vi "RT Main.vi"() -> ()   [LabVIEW 2019]
doc: "The myRIO Project template acquires acceleration data from the onboard accelerometer and displays the changes of acceleration values in a waveform chart."
uses:
  <vilib>/Platform/TimedLoop/XDataNode/timing_clust.ctl
  <vilib>/Platform/TimedLoop/XDataNode/nitl_modes.ctl
  <vilib>/Platform/TimedLoop/XDataNode/wakeup.ctl
  <vilib>/myRIO/Instrument Drivers/Onboard IO/AI/typedefs/AI Reference.ctl
  <vilib>/myRIO/Common/Instrument Driver Framework/Utilities/typedefs/myRIO Generic Hardware Reference.ctl
  <vilib>/myRIO/Common/Instrument Driver Framework/Utilities/typedefs/Hardware Version Enum.ctl
  <vilib>/myRIO/Common/Instrument Driver Framework/Utilities/typedefs/myRIO v1.0 Reference.ctl
  <vilib>/myRIO/Common/Instrument Driver Framework/Utilities/typedefs/Generic FPGA Reference.ctl
  <vilib>/myRIO/Common/Instrument Driver Framework/myRIO v1.0/AI/typedefs/AI Channels List.ctl
  <vilib>/myRIO/Common/Instrument Driver Framework/myRIO v1.0/AI/typedefs/AI Channels Enum.ctl
  <vilib>/myRIO/Common/Instrument Driver Framework/Utilities/typedefs/Analog Scaling Constants List.ctl
  <vilib>/myRIO/Common/Instrument Driver Framework/Utilities/typedefs/Analog Scaling Constants.ctl
  <vilib>/userDefined/High Color/nirio_resource_hc.ctl
  <vilib>/Simulation/Shared/_Datatypes/SIM SISO Transfer Function.ctl
  <vilib>/Analysis/Matrix/Datatypes/RealMatrix.ctl
  <vilib>/myRIO/Instrument Drivers/Onboard IO/AO/typedefs/AO Reference.ctl
  <vilib>/myRIO/Common/Instrument Driver Framework/myRIO v1.0/AO/typedefs/AO Channels List.ctl
  <vilib>/myRIO/Common/Instrument Driver Framework/myRIO v1.0/AO/typedefs/AO Channels Enum.ctl
  <vilib>/myRIO/Common/Instrument Driver Framework/Utilities/vis/Is FPGA Ref Available.vi
  <vilib>/myRIO/Common/Instrument Driver Framework/myRIO v1.0/AI/vis/myRIO v1.1 Open AI.vi
  <vilib>/myRIO/Instrument Drivers/Onboard IO/AI/vis/Read.vi
  <vilib>/Simulation/DiscreteLinear/Implementation/NILVSim Discrete Transfer Function Direct.llb/SIM Discrete Transfer Function Diagram (SISO).vi
  <vilib>/Analysis/7linalg.llb/Real Transpose Matrix.vi
  <vilib>/Analysis/baseanly.llb/Real A x B.vi
  <vilib>/myRIO/Common/Instrument Driver Framework/myRIO v1.0/AO/vis/myRIO v1.1 Open AO.vi
  <vilib>/myRIO/Instrument Drivers/Onboard IO/AO/vis/Write.vi
  <vilib>/myRIO/Common/Instrument Driver Framework/Utilities/vis/Validate Channels.vi
  <vilib>/myRIO/Common/Instrument Driver Framework/myRIO v1.0/AI/vis/myRIO v1.0 Reserve AI.vi
  <vilib>/Simulation/ContinuousLinear/Implementation/Shared/SIM Transfer Function Support.llb/SIM TransferFunction Normalize to Buffer.vi
  <vilib>/Simulation/DiscreteLinear/Implementation/Shared/SIM Init Discrete States.vi
  <vilib>/Simulation/DiscreteLinear/Implementation/NILVSim Discrete Transfer Function Direct.llb/SIM Transfer Function Direct core (SISO).vi
  <vilib>/myRIO/Common/Instrument Driver Framework/myRIO v1.0/AO/vis/myRIO v1.0 Reserve AO.vi
  <vilib>/myRIO/Common/Instrument Driver Framework/myRIO v1.0/AI/vis/myRIO v1.0 Build MUX Configuration AI.vi
  <vilib>/myRIO/Common/Instrument Driver Framework/myRIO v1.0/Resource Manager/vis/myRIO v1.0 Reserve Channel List.vi
  <vilib>/Simulation/ContinuousLinear/Implementation/Shared/SIM Transfer Function Support.llb/SIM TransferFunction Normalize.vi
  <vilib>/myRIO/Common/Instrument Driver Framework/myRIO v1.0/AO/vis/myRIO v1.0 Build MUX Configuration AO.vi
  <vilib>/myRIO/Common/Instrument Driver Framework/myRIO v1.0/Resource Manager/vis/myRIO v1.0 Reserve Channel.vi
  <vilib>/myRIO/Common/Instrument Driver Framework/myRIO v1.0/Resource Manager/vis/myRIO v1.0 Unreserve Channel.vi
  <vilib>/Simulation/Implementation/Shared/SIM Polynomials.llb/SIM Remove Zero Coefficients (DBL).vi
  <vilib>/myRIO/Common/Instrument Driver Framework/myRIO v1.0/Resource Manager/vis/myRIO v1.0 Build Mutex Name.vi
  <vilib>/Utility/VariantDataType/GetNumericInfo.vi
  <vilib>/Utility/error.llb/Error Cluster From Error Code.vi
  <vilib>/myRIO/Common/Instrument Driver Framework/myRIO v1.0/myRIO v1.1 Open.vi
  <vilib>/myRIO/Common/Instrument Driver Framework/myRIO v1.0/AI/vis/myRIO v1.0 Get Scaling Constants AI.vi
  <vilib>/myRIO/Common/Instrument Driver Framework/Utilities/vis/IO Manager.vi
  <vilib>/myRIO/Common/Instrument Driver Framework/Utilities/vis/Configuration Manager.vi
  <vilib>/myRIO/Common/Instrument Driver Framework/myRIO v1.0/myRIO v1.0 Close.vi
  <vilib>/myRIO/Common/Instrument Driver Framework/myRIO v1.0/AI/vis/myRIO v1.0 Read AI.vi
  <vilib>/Simulation/Implementation/Shared/SIM Polynomials.llb/SIM Divide Polynomials (DBL).vi
  <vilib>/Simulation/Implementation/Shared/SIM BuildSimErr.vi
  <vilib>/Analysis/Matrix/Numeric/Multiply/Multiply - R,RM.vi
  <vilib>/Analysis/Matrix/Numeric/Conversions/Array To Matrix - RA.vi
  <vilib>/myRIO/Common/Instrument Driver Framework/myRIO v1.0/AO/vis/myRIO v1.0 Get Scaling Constants AO.vi
  <vilib>/myRIO/Common/Instrument Driver Framework/myRIO v1.0/AO/vis/myRIO v1.0 Write AO.vi
  <vilib>/platform/TimedLoop/XDataNode/XDataNode.xnode
  <vilib>/myRIO/Express VI/Onboard IO/AI/AI Express VI.xnode
  <vilib>/myRIO/Instrument Drivers/Onboard IO/AI/vis/myRIO AI Open.xnode
  <vilib>/Simulation/Implementation/XNodeFramework/SimXNode/SimX.xnode
  <vilib>/myRIO/Express VI/Onboard IO/AO/AO Express VI.xnode
  <vilib>/myRIO/Instrument Drivers/Onboard IO/AO/vis/myRIO AO Open.xnode
  <vilib>/myRIO/Instrument Drivers/Onboard IO/AO/AO.lvlib
  <vilib>/Analysis/Matrix/NI_Matrix.lvlib
  <vilib>/myRIO/Instrument Drivers/Onboard IO/AI/AI.lvlib
  <vilib>/gmath/NI_Gmath.lvlib
  <vilib>/Analysis/NI_AALPro.lvlib
  <vilib>/Analysis/NI_AALBase.lvlib
  <vilib>/Platform/TimedLoop/XDataNode/XDNodeRunTimeDep.lvlib
  <vilib>/ptbypt/NI_PtbyPt.lvlib
panel:
  out "j data":dbl[](array[numeric])
  out "u data":dbl[](array[numeric])
  out "dx data":dbl[](array[numeric])
  out "x data":dbl[](array[numeric])
  out "sucess":bool
  in  "amplitude":dbl=0.0003
  out "imp":dbl
  out "Exitation":dbl(graph)
  out "dt":dbl=0.0005
  out "PD":bool
  out "J":dbl
  out "run time[s]":dbl
  out "t":dbl
  in  "max J":dbl=10.0
  out "control_law":string
  out "iterations":i32
  out "Last Cost (J)":dbl
  out "iteration duration":i64(graph)
  out "u[A]":dbl(graph)
  out "x[um]":dbl(graph)
  in  "Stop EM":bool=TRUE
  in  "Stop Button":bool
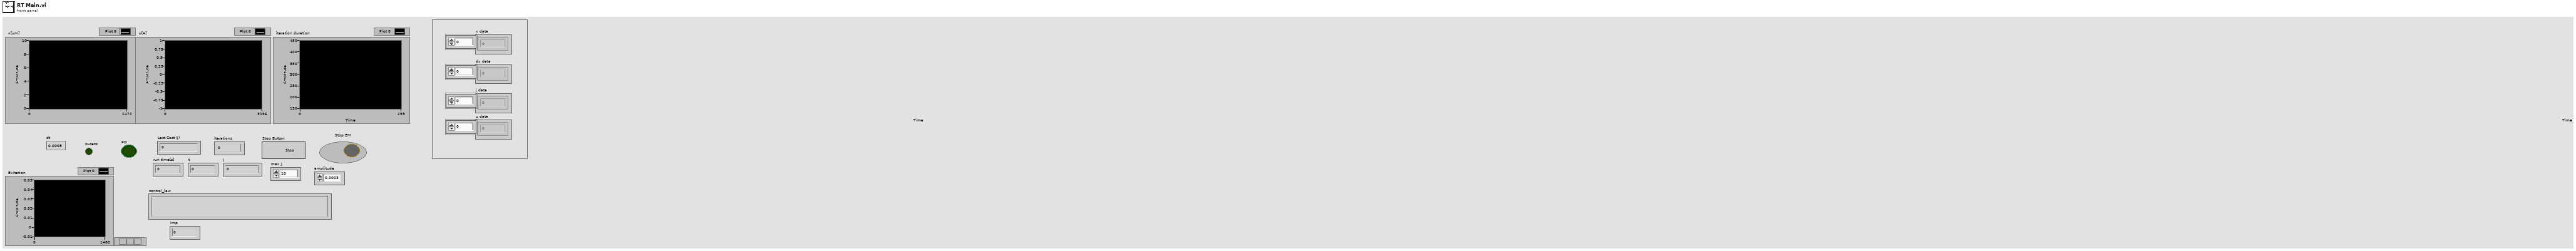
[diagram p1: front panel]
types:
  T1 = typedef "NI_Matrix.lvlib/RealMatrix.ctl" = dbl[][]
  T2 = typedef "SIM SISO Transfer Function.ctl" = cluster{"Numerator":dbl[], "Denominator":dbl[]}
  T3 = typedef "AO.lvlib/AO Reference.ctl" = cluster{"myRIO Reference":T4, "AO Channel List":T8, "AO Scaling Constant List":T10}
  T4 = typedef "myRIO Generic Hardware Reference.ctl" = cluster{"myRIO Model":T5, "myRIO Hardware Reference":T6}
  T5 = typedef "Hardware Version Enum.ctl" = enum16{"Unknown", "myRIO-1900", "myRIO-1950", "roboRIO", "NI ELVIS RIO CM", "ELVIS III"}
  T6 = typedef "myRIO v1.0 Reference.ctl" = cluster{"Generic FPGA Reference":T7, "Allow multiple opens":bool}
  T7 = typedef "Generic FPGA Reference.ctl" = refnum<k20>
  T8 = typedef "AO Channels List.ctl" = T9[]
  T9 = typedef "AO Channels Enum.ctl" = enum16{"Not Connected", "AudioOut/Left", "AudioOut/Right", "C/AO0", "C/AO1", "A/AO0", "A/AO1", "B/AO0", "B/AO1"}
  T10 = typedef "Analog Scaling Constants List.ctl" = T11[]
  T11 = typedef "Analog Scaling Constants.ctl" = cluster{"LSB Weight (Volts)":dbl, "Offset (Volts)":dbl, "Signed?":bool}
  T12 = typedef "nirio_resource_hc.ctl" = tag
  T13 = typedef "AI.lvlib/AI Reference.ctl" = cluster{"myRIO Reference":T4, "AI Channels List":T14, "AI Scaling Constants List":T10}
  T14 = typedef "AI Channels List.ctl" = T15[]
  T15 = typedef "AI Channels Enum.ctl" = enum16{"Not Connected", "AudioIn/Left", "AudioIn/Right", "C/AI0", "C/AI1", "A/AI0", "A/AI1", "A/AI2", "A/AI3", "A/AI4", "A/AI5", "A/AI6", "A/AI7", "B/AI0", "B/AI1", "B/AI2", "B/AI3", "B/AI4", "B/AI5", "B/AI6", "B/AI7", "AI/AI0", "AI/AI1", "AI/AI2", "AI/AI3", "A/AI0 (DIFF)", "A/AI1 (DIFF)", "A/AI2 (DIFF)", "A/AI3 (DIFF)", "B/AI0 (DIFF)", "B/AI1 (DIFF)", "B/AI2 (DIFF)", "B/AI3 (DIFF)"}
  T16 = typedef "XDNodeRunTimeDep.lvlib/timing_clust.ctl" = cluster{"Expected End [f-1]":u64, "Actual End [f-1]":u64, "Finished Late? [f-1]":bool, "Expected End [i-1]":u64, "Actual End [i-1]":u64, "Finished Late? [i-1]":bool, "Expected Start [i]":u64, "Actual Start [i]":u64, "Expected Start [f]":u64, "Actual Start [f]":u64, "Source Name":string, "Structure Name":string, "Period":i64, "Deadline":i64, "Offset":i64, "Start":i64, "Priority":i32, "Timeout":i32, "Mode":T17, "Wakeup Reason":T18, "Error":errorcluster, "Source Type":string, "Secondary Source Type":string, "Global End Time":u64, "Global Start Time":u64, "Frame Duration":u64, "Iteration Duration":u64, "Assigned CPU":i32, "I/O Scan Engine Mode":u32}
  T17 = typedef "XDNodeRunTimeDep.lvlib/nitl_modes.ctl" = enum32{"No Change", "Process missed periods, maintain original phase", "Discard missed periods, maintain original phase", "Process missed periods, ignore original phase", "Discard missed periods, ignore original phase"}
  T18 = typedef "XDNodeRunTimeDep.lvlib/wakeup.ctl" = enum32{"Normal", "Aborted", "Asynchronous wakeup", "Timing source error", "Timed loop error", "Timeout"}
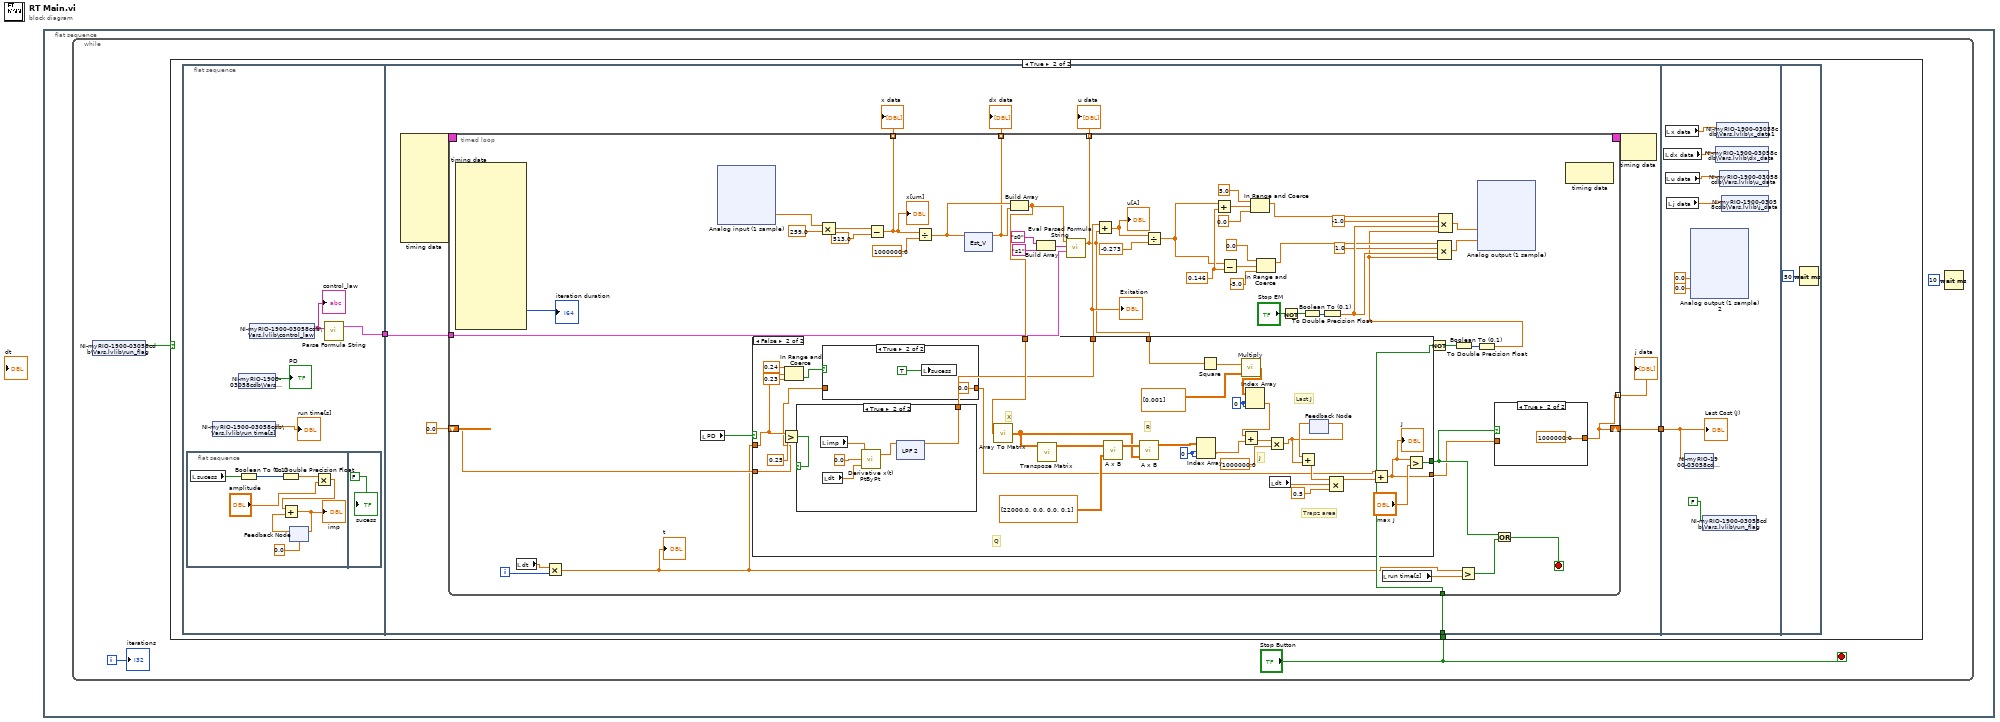
[diagram p0: block diagram]
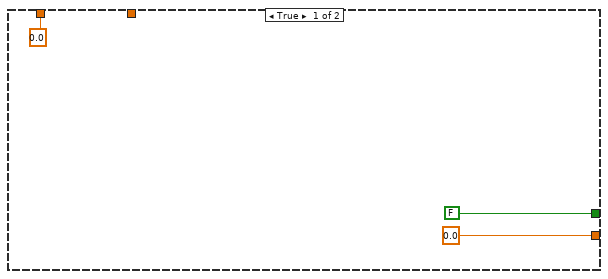
[diagram p4: hidden frame]
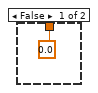
[diagram p6: hidden frame]
diagram:
  n1 = flat-sequence {
    frame #0 {
      n2 = while {
        i -> [w4]
        stop <- "Stop Button" stop-if-true
        n3 = shared-variable "NI-myRIO-1900-03058cdb\\Vars.lvlib\\run_flag"() -> (w2:bool)  [unwired: 1 in, 1 out]
        n4 = case shown="True" w2 {
          tunnel: "Stop Button" -> [_ w5]
          frame False {
          }
          frame True {
            n5 = flat-sequence {
              tunnel: [w10] -> w7
              tunnel: w7 -> [w28]
              tunnel: [w26] -> w6
              tunnel: w5 -> [w25]
              tunnel: w6 -> [w226]
              frame #0 {
                n6 = flat-sequence {
                  frame #0 {
                    n7 = local read "sucess"() -> (w17:bool)
                    n8 = Boolean To (0,1)(Boolean=w17) -> (0, 1=w18:i16)
                    n9 = To Double Precision Float(number=w18) -> (double precision float=w16:dbl)
                    n10 = feedback #1(0.0) -> (w19:dbl)
                    n11 = Multiply(x=w16, y="amplitude") -> (x*y=w12:dbl)
                    n12 = Add(x=w12, y=w19) -> (x+y=w13:dbl)
                    "imp" <- w13
                    n13 = feedback-in #1(w13) -> ()
                  }
                  frame #1 {
                    "sucess" <- FALSE ("sucess")
                  }
                }
                n14 = shared-variable "NI-myRIO-1900-03058cdb\\Vars.lvlib\\run time[s]"() -> (→"run time[s]":dbl)  [unwired: 1 in, 1 out]
                n15 = shared-variable "NI-myRIO-1900-03058cdb\\Vars.lvlib\\PD"() -> (→"PD":bool)  [unwired: 1 in, 1 out]
                n16 = shared-variable "NI-myRIO-1900-03058cdb\\Vars.lvlib\\control_law"() -> (w11:string)  [unwired: 1 in, 1 out]
                "control_law" <- w11
                n17 = call <vilib>:"Parse Formula String.vi"("formula"=w11) -> ("Parsed Formula"=w10:cluster{"Table":i32[][], "Y Values":dbl[]})  [unwired: 1 in, 1 out]
              }
              frame #1 {
                n18 = node-c288() -> (w30:T16)  [unwired: 10 in]
                n19 = timed-loop {
                  timing: w30 -> [_]
                  timing-out: [_] -> w29
                  shift-right: [w32] -> w26
                  shift-left: 0.0 -> [w59]
                  tunnel: w28 -> [w58]
                  tunnel: w25 -> [w41]
                  tunnel: [w35] -> w24 mode=indexing
                  tunnel: [w34] -> w23 mode=indexing
                  tunnel: [w33] -> w22 mode=indexing
                  tunnel: [w32] -> w21 mode=indexing
                  i -> [w47]
                  stop <- w44 stop-if-true
                  w75 = 0.146 ("y")
                  n20 = node-c288() -> (→"iteration duration":i64)  [unwired: 1 in, 16 out]
                  n21 = local read "dt"() -> (w31:dbl)
                  n22 = Multiply(x=w31, y=w47) -> (x*y=w37:dbl)
                  "t" <- w37
                  n23 = local read "PD"() -> (w43:bool)
                  n24 = xnode "Analog input (1 sample)"() -> ("C/AI1 (AI1)"=w64:dbl)  [unwired: 1 in, 1 out]
                  n25 = Multiply(x=w64, y=259.0) -> (x*y=w63:dbl)
                  n26 = Subtract(x=w63, y=513.0 ("x")) -> (x-y=w35:dbl)
                  "x[um]" <- w35
                  n27 = Divide(x=w35, y=1000000.0) -> (x/y=w46:dbl)
                  n28 = xnode "Est_V"("input u(k)"=w46) -> ("output y(k)"=w34:dbl)  [unwired: 2 in, 1 out]
                  n29 = Build Array(w46, w34) -> (w60:dbl[])
                  n30 = Build Array("s0", "s1") -> (w81:string[])
                  n31 = call <vilib>:"Eval Parsed Formula String.vi"("Parsed Formula"=w58, "Variables"=w81, "X Values"=w60) -> ("y value"=w33:dbl)  [unwired: 1 in, 1 out]
                  n32 = case shown="False" w43 {
                    tunnel: w60 -> [_ w118]
                    tunnel: w59 -> [_ w89]
                    tunnel: [0.0 w100] -> w39
                    tunnel: w33 -> [_ w104]
                    tunnel: [FALSE w103] -> w40
                    tunnel: w37 -> [_ w92]
                    tunnel: [0.0 w94] -> w36
                    frame True {
                    }
                    frame False {
                      w108 = 0 ("index (row)")
                      w109 = 0 ("disabled index (col)")
                      # "R"
                      # "Q"
                      # "J"
                      # "Trapz area"
                      # "Last J"
                      # "X"
                      n33 = Greater?(x=w92, y=0.25) -> (0:w95:bool)
                      n34 = In Range and Coerce(upper limit=0.24, x=w92, lower limit=0.23) -> (In Range?=w88:bool)  [unwired: 1 out]
                      n35 = case shown="True" w95 {
                        tunnel: [0.0 w126] -> w94
                        frame False {
                        }
                        frame True {
                          n36 = local read "imp"() -> (w125:dbl)
                          n37 = local read "dt"() -> (w127:dbl)
                          n38 = call <vilib>:"Derivative x(t) PtByPt.vi"("dt"=w127, "initial condition"=0.0, "x"=w125) -> ("dx/dt"=w128:dbl)  [unwired: 1 in, 1 out]
                          n39 = xnode "LPF 2"("input u(k)"=w128) -> ("output y(k)"=w126:dbl)  [unwired: 2 in, 1 out]
                        }
                      }
                      n40 = case shown="True" w88 {
                        tunnel: w89 -> [w121 _]
                        tunnel: [w121 0.0] -> w87
                        frame False {
                        }
                        frame True {
                          n41 = local write "sucess"(TRUE) -> ()
                        }
                      }
                      n42 = call-poly <vilib>:"Array To Matrix.vi"("Real 1D Array"=w118) -> ("Real Matrix (Column Vector)"=w116:T1)
                      n43 = call-poly <vilib>:"Transpose Matrix.vi"("Input Matrix"=w116) -> ("Matrix Transpose"=w120:T1)  [unwired: 9 in, 1 out]
                      n44 = call-poly <vilib>:"A x B.vi"("B"=T1 [[22000.0, 0.0], [0.0, 0.1]], "A"=w120) -> ("A x B"=w119:T1)  [unwired: 1 out]
                      n45 = call-poly <vilib>:"A x B.vi"("B"=w116, "A"=w119) -> ("A x B"=w112:T1)  [unwired: 1 out]
                      n46 = Index Array(array=w112, index (row)=w108, index (col)=w108) -> (element=w111:dbl)
                      n47 = Square(x=w104) -> (x^2=w117:dbl)
                      n48 = call-poly <vilib>:"Multiply.vi"("Real Matrix A"=T1 [[0.001]], "Real Scalar c"=w117) -> ("c * A"=w114:T1)
                      n49 = Index Array(array=w114, index (row)=w109, index (col)=w109) -> (element=w113:dbl)
                      n50 = Add ("Add.vi")(x=w113, y=w111) -> (x+y=w99:dbl)
                      n51 = Multiply ("Multiply.vi")(x=w99, y=1000000.0) -> (x*y=w97:dbl)
                      n52 = local read "dt"() -> (w93:dbl)
                      n53 = feedback #2() -> (w115:dbl)  [unwired: 1 in]
                      n54 = Add ("Add.vi")(x=w115, y=w97) -> (x+y=w107:dbl)
                      n55 = feedback-in #2(w97) -> ()
                      n56 = Compound Arithmetic op=MULTIPLY(w107, w93, 0.5 ("value")) -> (w105:dbl)
                      n57 = Add ("Add.vi")(x=w87, y=w105) -> (x+y=w100:dbl)
                      "J" <- w100
                      n58 = Greater?(x=w100, y="max J") -> (0:w103:bool)
                    }
                  }
                  "Exitation" <- w36
                  n59 = Add(x=w36, y=w33) -> (x+y=w38:dbl)
                  "u[A]" <- w38
                  n60 = Divide(x=w38, y=-0.273) -> (x/y=w74:dbl)
                  n61 = Add(x=w74, y=w75) -> (x+y=w73:dbl)
                  n62 = Subtract(x=w74, y=w75) -> (x-y=w72:dbl)
                  n63 = In Range and Coerce(upper limit=5.0, x=w73, lower limit=0.0) -> (coerced(x)=w55:dbl)  [unwired: 1 out]
                  n64 = In Range and Coerce(upper limit=0.0, x=w72, lower limit=-5.0) -> (coerced(x)=w50:dbl)  [unwired: 1 out]
                  n65 = Not(x="Stop EM") -> (.not. x?=w66:bool)
                  n66 = Boolean To (0,1)(Boolean=w66) -> (0, 1=w65:i16)
                  n67 = To Double Precision Float(number=w65) -> (double precision float=w52:dbl)
                  n68 = local read "run time[s]"() -> (w42:dbl)
                  n69 = Not(x=w41) -> (.not. x?=w57:bool)
                  n70 = Boolean To (0,1)(Boolean=w57) -> (0, 1=w56:i16)
                  n71 = Greater?(x=w37, y=w42) -> (0:w45:bool)
                  n72 = To Double Precision Float(number=w56) -> (double precision float=w49:dbl)
                  n73 = Compound Arithmetic op=MULTIPLY(w50, 1.0 ("value"), w52, w49) -> (w48:dbl)
                  n74 = Compound Arithmetic op=MULTIPLY(w55, -1.0 ("value"), w52, w49) -> (w53:dbl)
                  n75 = xnode "Analog output (1 sample)"("C/AO0 (AO0)"=w53, "C/AO1 (AO1)"=w48) -> ()  [unwired: 1 in, 1 out]
                  n76 = case shown="True" w40 {
                    tunnel: [w82 1000000.0] -> w32
                    tunnel: w39 -> [w82 _]
                    frame False {
                    }
                    frame True {
                    }
                  }
                  n77 = Or(x=w40, y=w45) -> (x .or. y?=w44:bool)
                  n78 = node-c288() -> ()  [unwired: 1 in, 1 out]
                }
                "x data" <- w24
                "dx data" <- w23
                "u data" <- w22
                "j data" <- w21
                n79 = node-c288(w29) -> ()  [unwired: 1 out]
              }
              frame #2 {
                n80 = local read "dx data"() -> (w224:dbl[])
                n81 = local read "x data"() -> (w225:dbl[])
                n82 = local read "u data"() -> (w222:dbl[])
                n83 = local read "j data"() -> (w223:dbl[])
                n84 = shared-variable "NI-myRIO-1900-03058cdb\\Vars.lvlib\\J"(w226) -> ()  [unwired: 1 in, 1 out]
                n85 = xnode "Analog output (1 sample) 2"("C/AO0 (AO0)"=0.0, "C/AO1 (AO1)"=0.0) -> ()  [unwired: 1 in, 1 out]
                n86 = shared-variable "NI-myRIO-1900-03058cdb\\Vars.lvlib\\run_flag"(FALSE ("run_flag")) -> ()  [unwired: 1 in, 1 out]
                n87 = shared-variable "NI-myRIO-1900-03058cdb\\Vars.lvlib\\dx_data"(w224) -> ()  [unwired: 1 in, 1 out]
                n88 = shared-variable "NI-myRIO-1900-03058cdb\\Vars.lvlib\\x_data1"(w225) -> ()  [unwired: 1 in, 1 out]
                n89 = shared-variable "NI-myRIO-1900-03058cdb\\Vars.lvlib\\u_data"(w222) -> ()  [unwired: 1 in, 1 out]
                n90 = shared-variable "NI-myRIO-1900-03058cdb\\Vars.lvlib\\j_data"(w223) -> ()  [unwired: 1 in, 1 out]
                "Last Cost (J)" <- w226
              }
              frame #3 {
                n91 = Wait (ms)(milliseconds to wait=u32 50) -> ()  [unwired: 1 out]
              }
            }
          }
        }
        n92 = Wait (ms)(milliseconds to wait=u32 10) -> ()  [unwired: 1 out]
        "iterations" <- w4
      }
    }
  }
